vi "Staib EG Bk.vi"(0 "Computer\nControl":bool, 1 "Energy (eV)":dbl(knob) min=0.0 max=100.0 step=0.001 scale=0.0..100.0 scale format="%#_3g", 3 "Extraction (V)":dbl(knob) min=0.0 max=100.0 step=0.001 scale=0.0..100.0 scale format="%#_3g", 4 "Filament (V)":dbl(knob) min=0.0 max=10.0 step=0.001 scale=0.0..5.0 scale format="%#_3g", 5 "Grid (V)":dbl(knob) min=-15.0 max=15.0 step=0.001 scale=-15.0..15.0 scale format="%#_3g", 6 "Focus 1 (V)":dbl(knob) min=-0.0 max=0.0 step=0.001 scale=0.0..1.0 scale format="%#_3g", 8 "error in":errorcluster, 10 "Focus 2 (V)":dbl(knob) min=-0.0 max=0.0 step=0.001 scale=0.0..1.0 scale format="%#_3g", 12 "Lock Focus":bool, 14 "X1 Alignment (V)":dbl(knob) min=-10.0 max=10.0 step=0.001 scale=-10.0..10.0 scale format="%#_3g", 15 "X2 Alignment (V)":dbl(knob) min=-10.0 max=10.0 step=0.001 scale=-10.0..10.0 scale format="%#_3g", 17 "Y1 Alignment (V)":dbl(knob) min=-10.0 max=10.0 step=0.001 scale=-10.0..10.0 scale format="%#_3g", 18 "Y2 Alignment (V)":dbl(knob) min=-10.0 max=10.0 step=0.001 scale=-10.0..10.0 scale format="%#_3g") -> (7 "Focus Min (V)":dbl, 9 "error out":errorcluster, 11 "Focus Max (V)":dbl min=0.0 max=100.0 step=0.001, 13 "Focus Disable":i32, 19 "Computer\nControl Enabled?":bool)   [LabVIEW 2010]
uses:
  <vilib>/DAQmx/write.llb/DAQmx Write (Analog DBL 1Chan 1Samp).vi
  <vilib>/DAQmx/write.llb/DAQmx Write (Digital Bool 1Line 1Point).vi
  <vilib>/daqmx/miscellaneous.llb/DAQmx Fill In Error Info.vi
panel:
  # "On"
  # "Off"
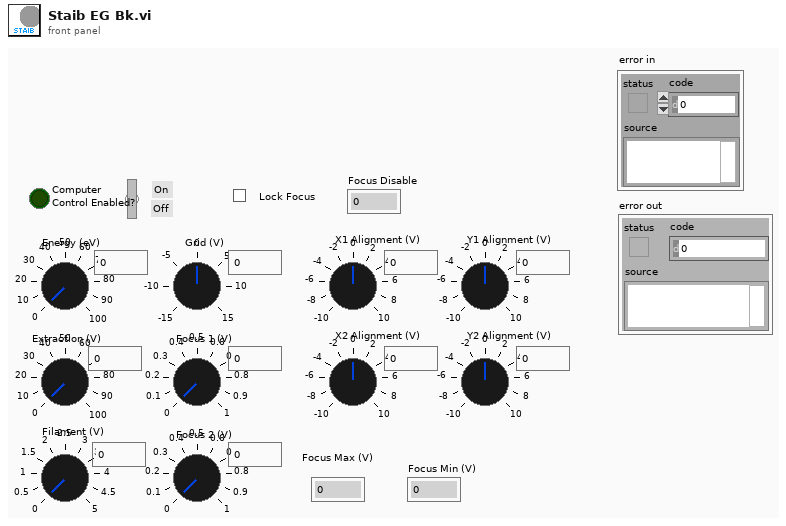
[diagram p1: front panel]
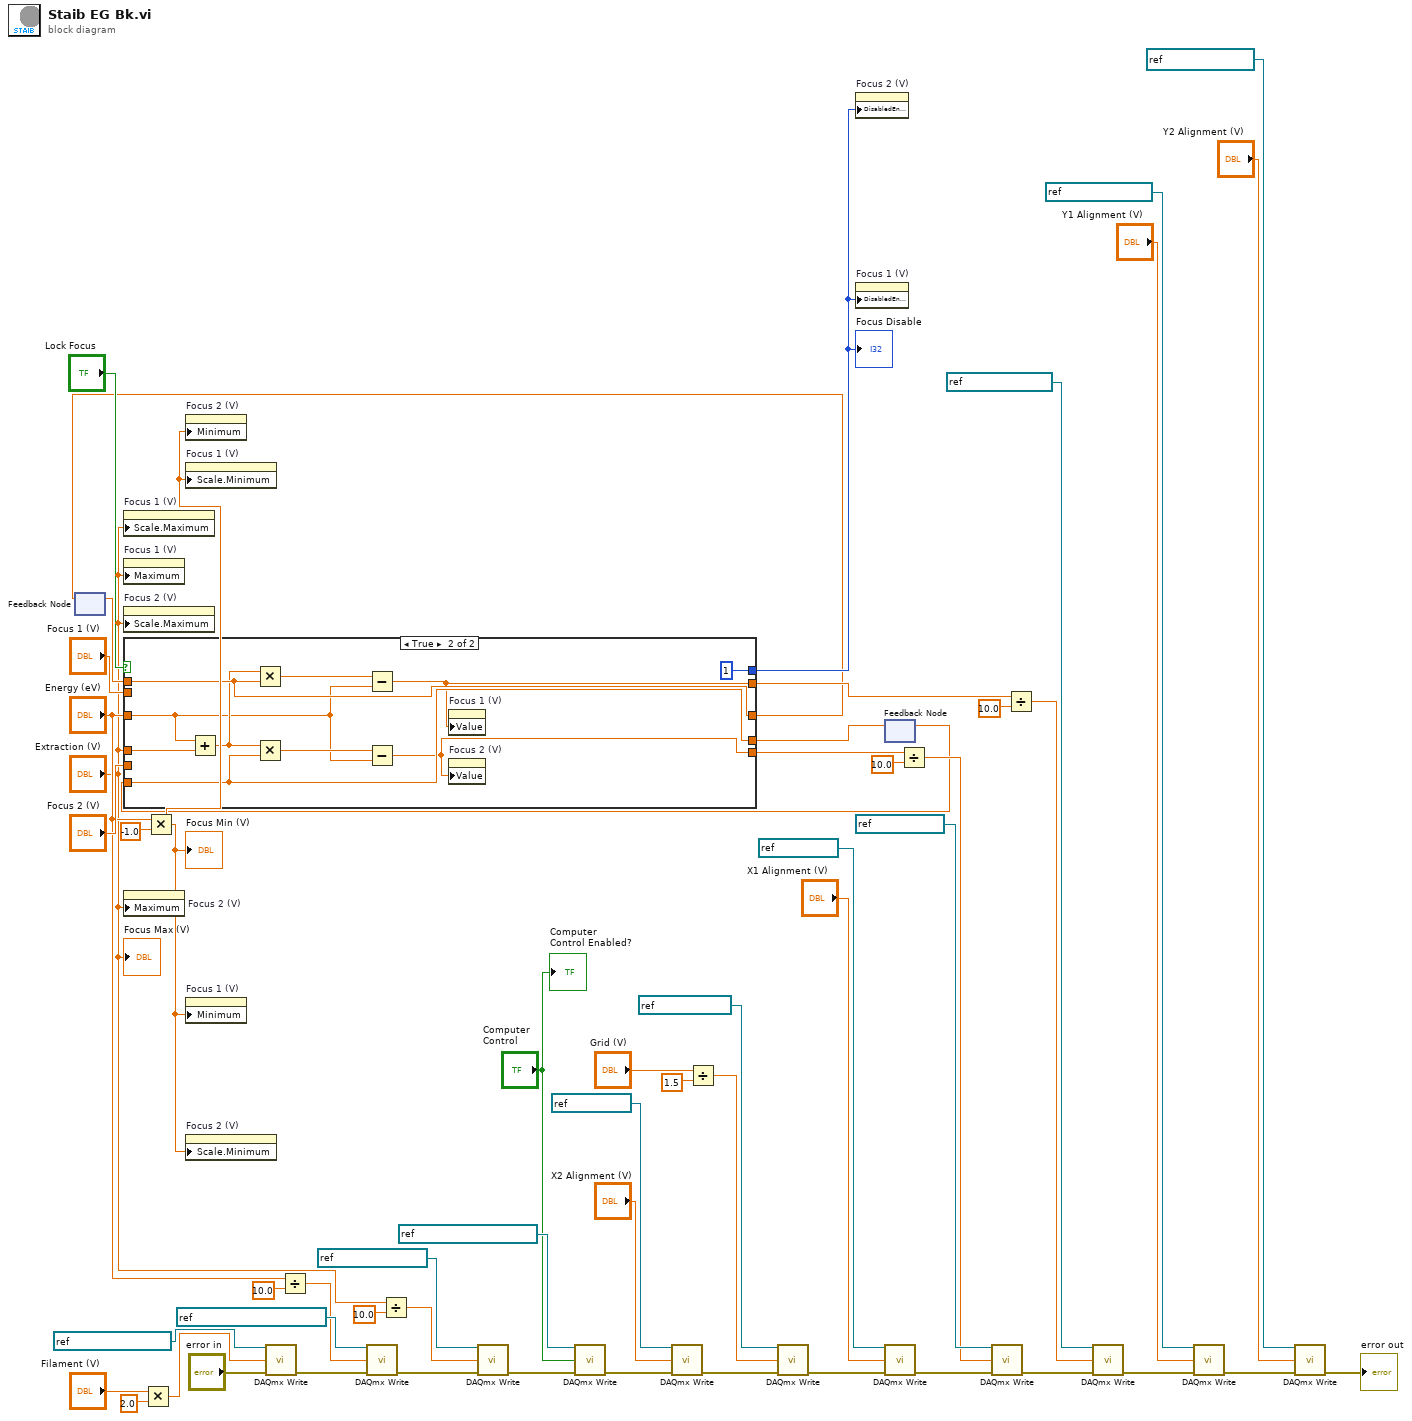
[diagram p0: block diagram]
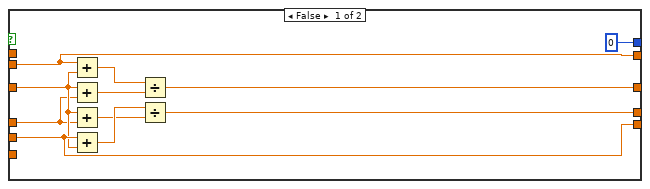
[diagram p2: hidden frame]
diagram:
  n1 = feedback #1() -> (w17:dbl)  [unwired: 1 in]
  n2 = property on="Focus 1 (V)" class="Knob (strict)"("Scale.Maximum"="Extraction (V)") -> ()  [unwired: 2 in, 2 out]
  n3 = property on="Focus 1 (V)" class="Knob (strict)"("Maximum"="Extraction (V)") -> ()  [unwired: 2 in, 2 out]
  n4 = property on="Focus 2 (V)" class="Knob (strict)"("Scale.Maximum"="Extraction (V)") -> ()  [unwired: 2 in, 2 out]
  n5 = property on="Focus 2 (V)" class="Knob (strict)"("Maximum"="Extraction (V)") -> ()  [unwired: 2 in, 2 out]
  n6 = Multiply(x="Filament (V)", y=2.0) -> (x*y=w37:dbl)
  n7 = Multiply(x="Energy (eV)", y=-1.0) -> (x*y=w30:dbl)
  "Focus Min (V)" <- w30
  n8 = property on="Focus 2 (V)" class="Knob (strict)"("Minimum"=w30) -> ()  [unwired: 2 in, 2 out]
  n9 = property on="Focus 1 (V)" class="Knob (strict)"("Scale.Minimum"=w30) -> ()  [unwired: 2 in, 2 out]
  n10 = property on="Focus 1 (V)" class="Knob (strict)"("Minimum"=w30) -> ()  [unwired: 2 in, 2 out]
  n11 = property on="Focus 2 (V)" class="Knob (strict)"("Scale.Minimum"=w30) -> ()  [unwired: 2 in, 2 out]
  n12 = call-poly <vilib>:"DAQmx Write.vi"("task/channels in"=refnum<k21> "Filament out", "data"=w37, "error in"="error in") -> ("error out"=w12:errorcluster)  [unwired: 10 in, 2 out]
  n13 = Divide(x="Energy (eV)", y=10.0) -> (x/y=w33:dbl)
  n14 = call-poly <vilib>:"DAQmx Write.vi"("task/channels in"=refnum<k21> "Electron Energy Out", "data"=w33, "error in"=w12) -> ("error out"=w11:errorcluster)  [unwired: 10 in, 2 out]
  n15 = Divide(x="Extraction (V)", y=10.0) -> (x/y=w39:dbl)
  n16 = call-poly <vilib>:"DAQmx Write.vi"("task/channels in"=refnum<k21> "Extraction out", "data"=w39, "error in"=w11) -> ("error out"=w10:errorcluster)  [unwired: 10 in, 2 out]
  n17 = call-poly <vilib>:"DAQmx Write.vi"("task/channels in"=refnum<k21> "ElectronCPUControl", "data"="Computer\nControl", "error in"=w10) -> ("error out"=w9:errorcluster)  [unwired: 10 in, 2 out]
  n18 = call-poly <vilib>:"DAQmx Write.vi"("task/channels in"=refnum<k21> "X2 out", "data"="X2 Alignment (V)", "error in"=w9) -> ("error out"=w8:errorcluster)  [unwired: 10 in, 2 out]
  n19 = Divide(x="Grid (V)", y=1.5) -> (x/y=w42:dbl)
  n20 = call-poly <vilib>:"DAQmx Write.vi"("task/channels in"=refnum<k21> "Grid Out", "data"=w42, "error in"=w8) -> ("error out"=w7:errorcluster)  [unwired: 10 in, 2 out]
  n21 = feedback #2() -> (w15:dbl)  [unwired: 1 in]
  n22 = case shown="True" "Lock Focus" {
    tunnel: "Focus 2 (V)" -> [w60 _]
    tunnel: [w60 w68] -> w20
    tunnel: "Focus 1 (V)" -> [w66 _]
    tunnel: [w66 w69] -> w22
    tunnel: [0 1] -> w25
    tunnel: "Energy (eV)" -> [w59 w70]
    tunnel: "Extraction (V)" -> [w58 w76]
    tunnel: [w63 w74] -> w18
    tunnel: [w57 w72] -> w16
    tunnel: w17 -> [_ w74]
    tunnel: w15 -> [_ w72]
    frame False {
      n23 = Add(x=w66, y=w59) -> (x+y=w65:dbl)
      n24 = Add(x=w59, y=w58) -> (x+y=w64:dbl)
      n25 = Add(x=w59, y=w58) -> (x+y=w61:dbl)
      n26 = Add(x=w60, y=w59) -> (x+y=w62:dbl)
      n27 = Divide(x=w65, y=w64) -> (x/y=w63:dbl)
      n28 = Divide(x=w62, y=w61) -> (x/y=w57:dbl)
    }
    frame True {
      n29 = Add(x=w70, y=w76) -> (x+y=w73:dbl)
      n30 = Multiply(x=w73, y=w74) -> (x*y=w75:dbl)
      n31 = Multiply(x=w73, y=w72) -> (x*y=w71:dbl)
      n32 = Subtract(x=w75, y=w70) -> (x-y=w69:dbl)
      n33 = Subtract(x=w71, y=w70) -> (x-y=w68:dbl)
      n34 = property on="Focus 1 (V)" class="Knob (strict)"("Value"=w69) -> ()  [unwired: 2 in, 2 out]
      n35 = property on="Focus 2 (V)" class="Knob (strict)"("Value"=w68) -> ()  [unwired: 2 in, 2 out]
    }
  }
  "Focus Disable" <- w25
  n36 = feedback-in #1(w18) -> ()
  n37 = property on="Focus 2 (V)" class="Knob (strict)"("DisabledEnum"=w25) -> ()  [unwired: 2 in, 2 out]
  n38 = property on="Focus 1 (V)" class="Knob (strict)"("DisabledEnum"=w25) -> ()  [unwired: 2 in, 2 out]
  n39 = feedback-in #2(w16) -> ()
  n40 = call-poly <vilib>:"DAQmx Write.vi"("task/channels in"=refnum<k21> "X1 out", "data"="X1 Alignment (V)", "error in"=w7) -> ("error out"=w6:errorcluster)  [unwired: 10 in, 2 out]
  n41 = Divide(x=w20, y=10.0) -> (x/y=w27:dbl)
  n42 = call-poly <vilib>:"DAQmx Write.vi"("task/channels in"=refnum<k21> "Focus 2 out", "data"=w27, "error in"=w6) -> ("error out"=w5:errorcluster)  [unwired: 10 in, 2 out]
  n43 = Divide(x=w22, y=10.0) -> (x/y=w24:dbl)
  n44 = call-poly <vilib>:"DAQmx Write.vi"("task/channels in"=refnum<k21> "Focus 1 out", "data"=w24, "error in"=w5) -> ("error out"=w4:errorcluster)  [unwired: 10 in, 2 out]
  n45 = call-poly <vilib>:"DAQmx Write.vi"("task/channels in"=refnum<k21> "Y1 out", "data"="Y1 Alignment (V)", "error in"=w4) -> ("error out"=w3:errorcluster)  [unwired: 10 in, 2 out]
  n46 = call-poly <vilib>:"DAQmx Write.vi"("task/channels in"=refnum<k21> "Y2 out", "data"="Y2 Alignment (V)", "error in"=w3) -> ("error out"=→"error out":errorcluster)  [unwired: 10 in, 2 out]
  "Computer\nControl Enabled?" <- "Computer\nControl"
  "Focus Max (V)" <- "Extraction (V)"
